vi "SV- Command.vi"(8 "error in (no error)":errorcluster, 11 "PSP-405 resource in":refnum<visa-resource-name>) -> (0 "error out":errorcluster, 3 "PSP-405 resource out":refnum<visa-resource-name>)   [LabVIEW 2017, in "GW Instek PSP-405.lvlib"]
doc: "The SV- command decreases the voltage output by 1V (coarse mode) or 1mV (fine mode). \nExample:\n20.00V › 19.00V (coarse mode) \n20.00V › 19.99V (fine mode)"
uses:
  GW Instek PSP-405.lvlib
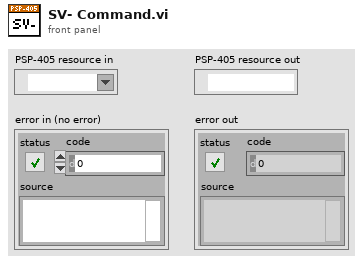
[diagram p1: front panel]
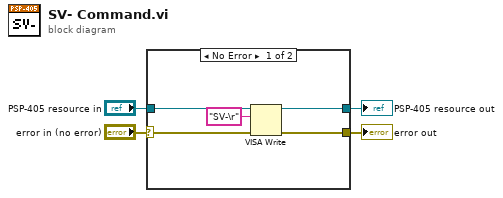
[diagram p0: block diagram]
diagram:
  n1 = case shown="No Error" "error in (no error)" {
    selector: "error in (no error)" -> [w6 w11]
    tunnel: "PSP-405 resource in" -> [w8 w10]
    tunnel: [w9 w11] -> w3
    tunnel: [w5 w10] -> w1
    frame No Error {
      n2 = VISA Write(VISA resource name=w8, write buffer="SV-\r" ("cmd"), error in (no error)=w6) -> (VISA resource name out=w5:refnum<visa-resource-name>, error out=w9:errorcluster)  [unwired: 1 out]
    }
    frame Error {
    }
  }
  "error out" <- w3
  "PSP-405 resource out" <- w1
